vi "Cluster Variant to Key List.vi"(5 "section":string, 7 "Prefix":string, 8 "Error In":errorcluster, 11 "Variant":variant) -> (0 "Error Out":errorcluster, 2 "Key list":T1)   [LabVIEW 2015]
uses:
  <vilib>/Utility/Data Type/NI_Data Type.lvlib
panel:
  in  "Number of elements":i32
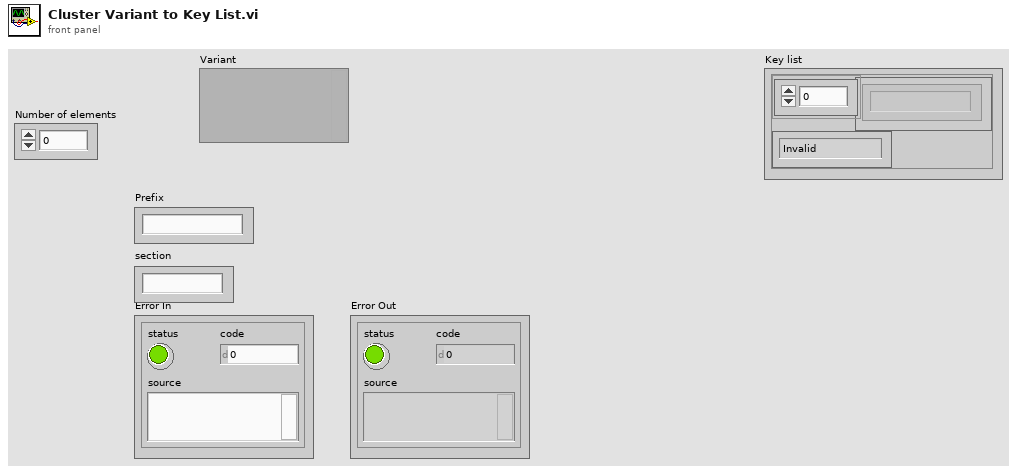
[diagram p1: front panel]
types:
  T1 = cluster{"Array":string[], "Enum":enum16{"Invalid", "Boolean", "Double", "I32", "Path", "String", "U32", "Array", "Cluster"}}
  T2 = enum16{"Invalid", "Boolean", "Double", "I32", "Path", "String", "U32", "Array", "Cluster"}
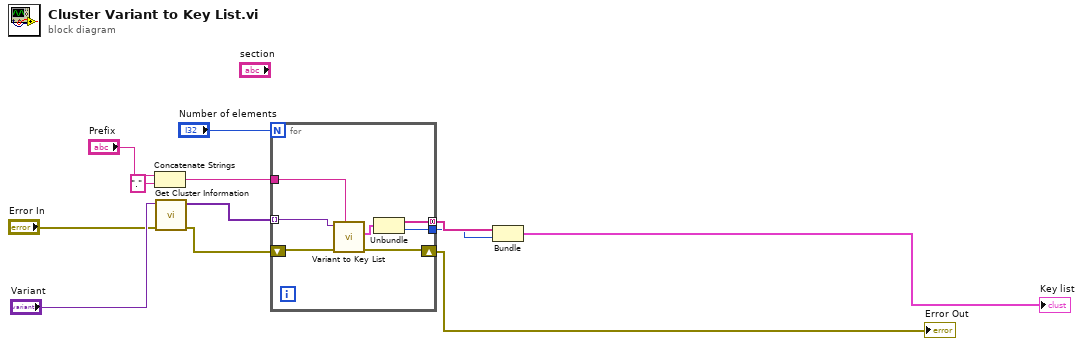
[diagram p0: block diagram]
diagram:
  n1 = Concatenate Strings("Prefix", "." ("string")) -> (w5:string)
  n2 = call <vilib>:"Get Cluster Information.vi"("error in (no error)"="Error In", "Variant"="Variant") -> ("error out"=w7:errorcluster, "Cluster Elements"=w8:variant[])  [unwired: 8 in]
  n3 = for {
    N: "Number of elements" -> [_]
    tunnel: w8 -> [w19] mode=indexing
    shift-right: [w16] -> w1
    shift-left: w7 -> [w17]
    tunnel: w5 -> [w18]
    tunnel: [w14] -> w4 mode=concatenating
    tunnel: [w13] -> w3
    n4 = call "Variant to Key List.vi"("Prefix"=w18, "Error In"=w17, "Variant"=w19) -> ("Error Out"=w16:errorcluster, "Key list"=w15:T1)  [unwired: 7 in]
    n5 = Unbundle(w15) -> ("Array"=w14:string[], "Enum"=w13:T2)
  }
  "Error Out" <- w1
  n6 = Bundle("Array"=w4, "Enum"=w3) -> (→"Key list":T1)  [unwired: 1 in]
